vi "daq_TL Motor3DScan_initial2.vi"() -> ()   [LabVIEW 2014]
doc: "2D motor scan example Vi."
panel:
  in  "Z0 (33)":sgl format="%.3f"
  in  "X0 (34)":sgl=8.1 format="%.3f"
  in  "Y0 (32)":sgl=7.5 format="%.3f"
  out "Picture":picture
  out "Scale Z":sgl=0.1 format="%.3f"
  in  "Num Of Steps Z":i32=2
  out "MG17Motor C":dbl
  in  "Channel C":i32
  in  "Motor HWSerialNum C":u32=90834933
  in  "MG17Motor C":refnum<k7>(container)
  out "unsigned 8bit integer":u8[][](array[numeric])
  out "DAQ":dbl[][](array[numeric])
  out "Y":dbl[](array[numeric])
  out "Waveform Graph":waveform(dbl)(graph)
  out "dt":dbl
  out "t0":timestamp
  out "MG17Motor A":dbl
  out "MG17Motor B":dbl
  in  "Motor HWSerialNum B":u32=90834934
  in  "MG17Motor B":refnum<k7>(container)
  in  "MG17Motor A":refnum<k7>(container)
  in  "Num Of Steps X Y":i32=2
  out "Scale X Y":sgl=0.1 format="%.3f"
  in  "Both Channels":i32=10
  in  "Channel B":i32
  in  "Channel A":i32
  out "error":errorcluster
  in  "Motor HWSerialNum A":u32=90834932
  # "MG17Motor B\n (Y)"
  # "MG17Motor A\n (X)"
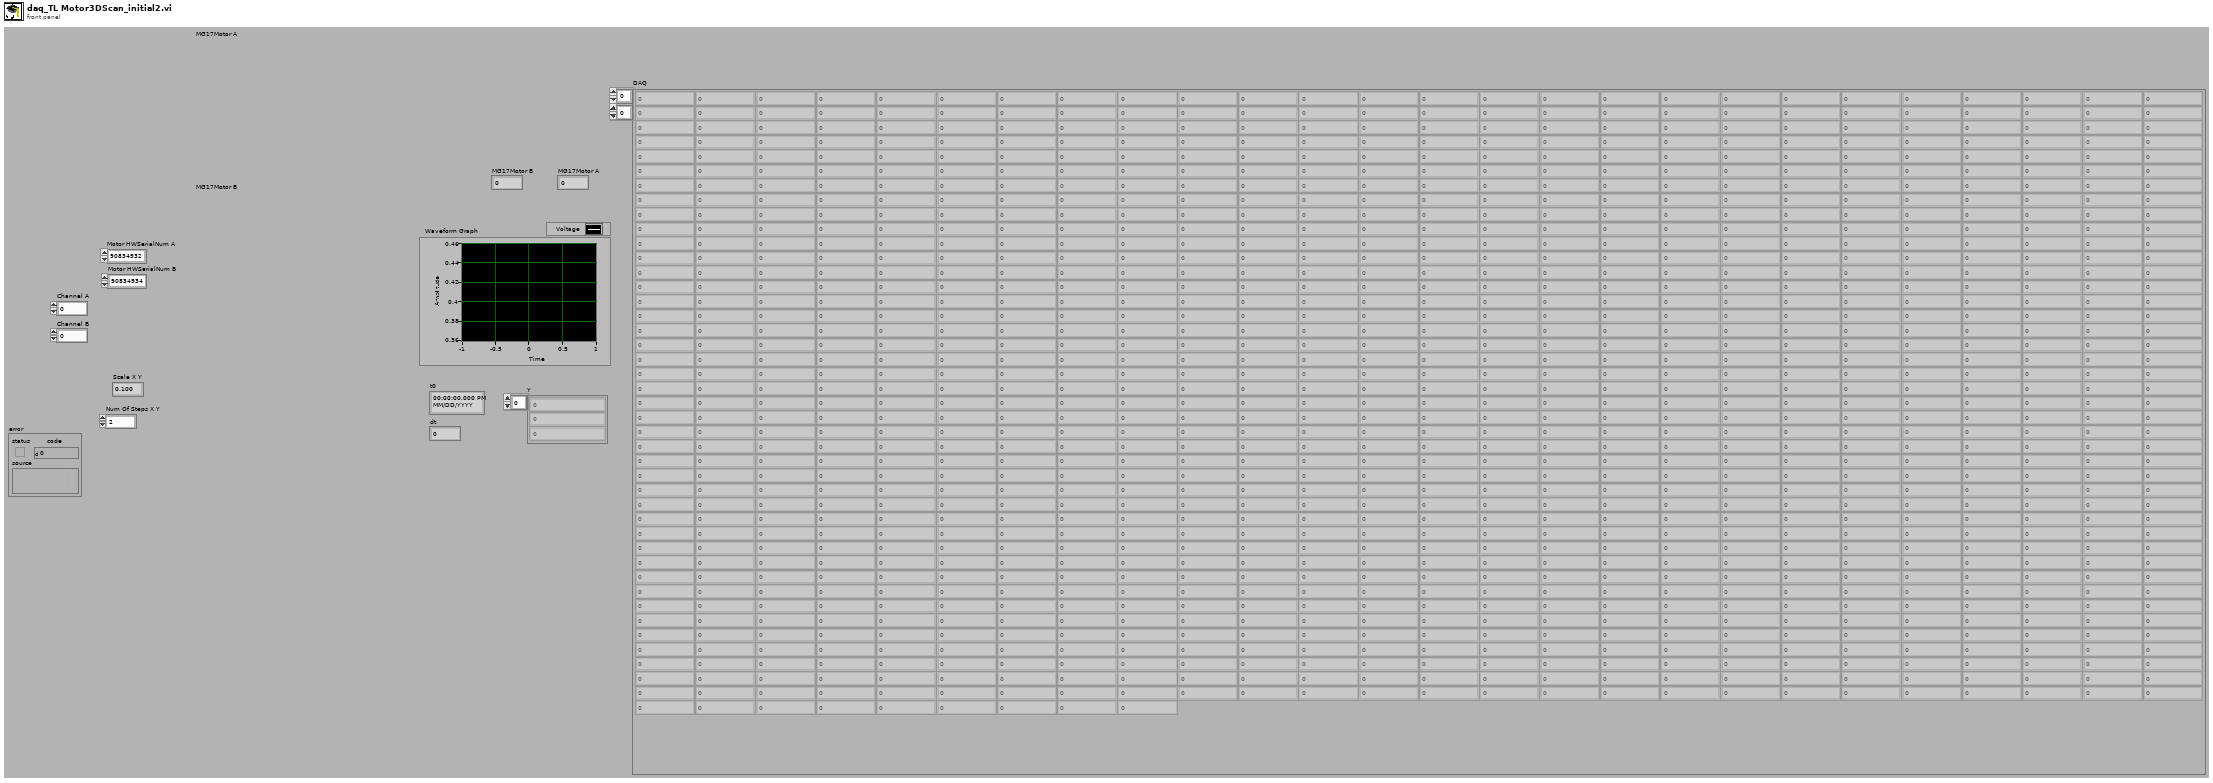
[diagram p1: front panel]
types:
  T1 = typedef "imagedata.ctl" = cluster{"image type":i32, "image depth":i32, "image":u8[], "mask":u8[], "colors":u32[], "Rectangle":cluster{"left":i16, "top":i16, "right":i16, "bottom":i16}}
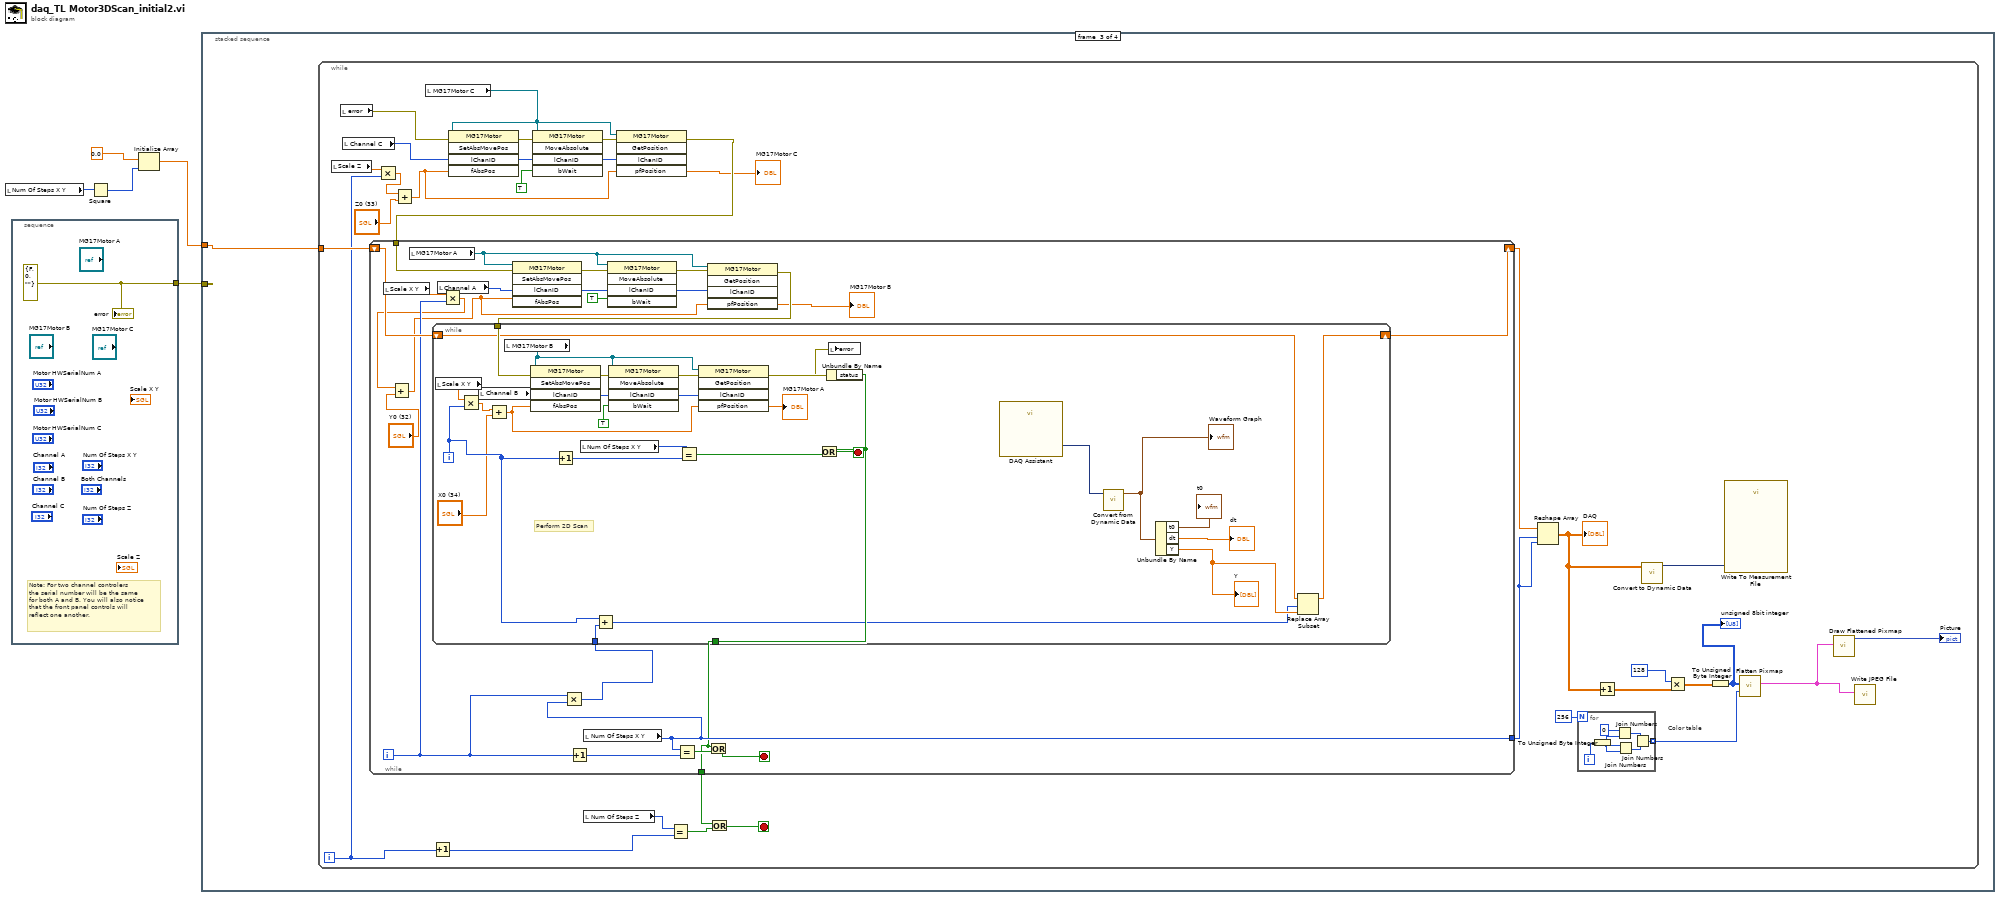
[diagram p0: block diagram]
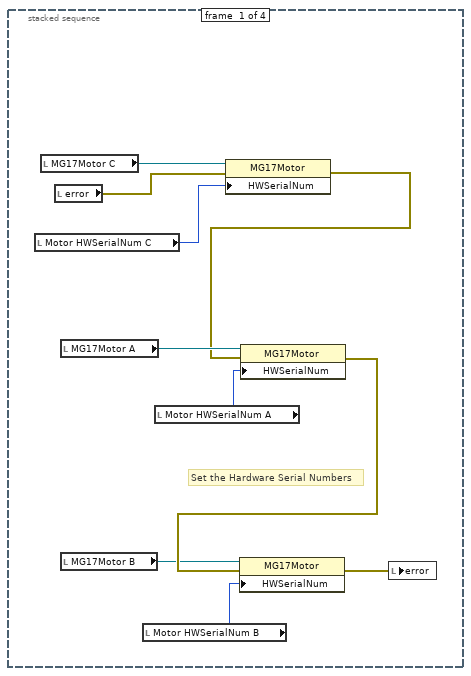
[diagram p2: hidden frame]
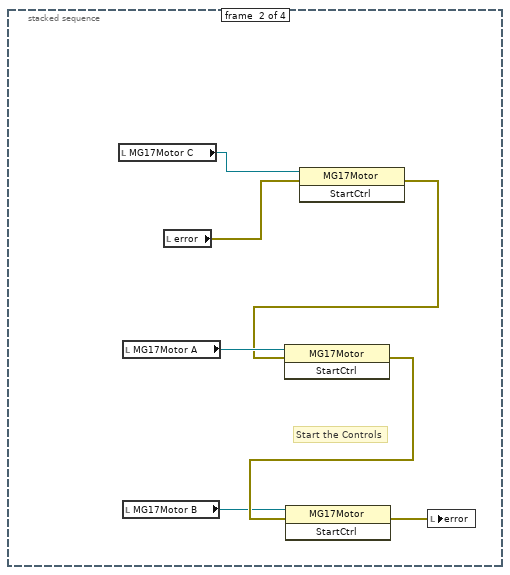
[diagram p3: hidden frame]
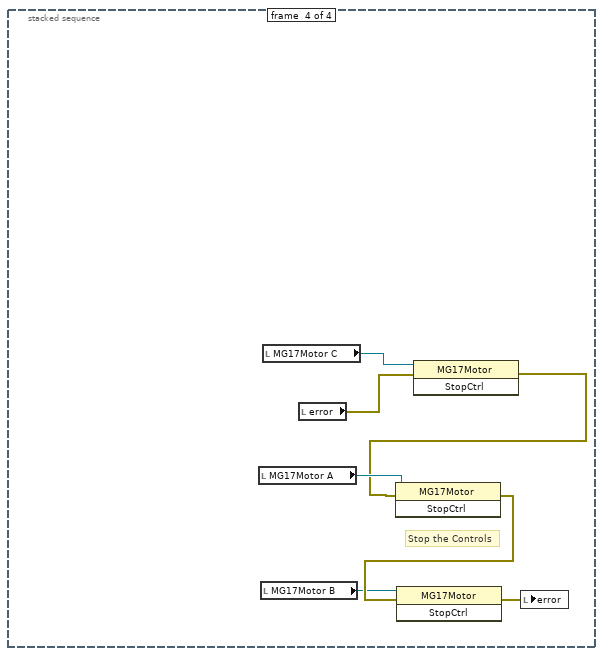
[diagram p4: hidden frame]
diagram:
  n1 = local read "Num Of Steps X Y"() -> (w1:i32)
  n2 = stacked-sequence {
    tunnel: [w6] -> w5
    frame #0 {
      w6 = errorcluster {"status"=FALSE, "code"=0, "source"=""} ("error in (no error)")
      # "Note: For two channel controlers\nthe serial number will be the same\nfor both A and B. You will also notice\nthat the front panel controls will\nreflect one another."
      "error" <- w6
    }
  }
  n3 = Square(x=w1) -> (x^2=w2:i32)
  n4 = Initialize Array(0.0, w2) -> (w3:dbl[])
  n5 = stacked-sequence {
    tunnel: w5 -> [_ _ _ _]
    tunnel: w3 -> [_ _ w24 _]
    frame #0 {
      # "Set the Hardware Serial Numbers"
      n6 = local read "Motor HWSerialNum C"() -> (w7:u32)
      n7 = local read "MG17Motor C"() -> (w10:refnum<k7>)
      n8 = local read "error"() -> (w9:errorcluster)
      n9 = local read "MG17Motor A"() -> (w15:refnum<k7>)
      n10 = local read "MG17Motor B"() -> (w12:refnum<k7>)
      n11 = local read "Motor HWSerialNum B"() -> (w11:u32)
      n12 = local read "Motor HWSerialNum A"() -> (w16:u32)
      n13 = property class="MG17Motor"(reference=w10, error in=w9, "HWSerialNum"=w7) -> (error out=w8:errorcluster)  [unwired: 1 out]
      n14 = property class="MG17Motor"(reference=w15, error in=w8, "HWSerialNum"=w16) -> (error out=w14:errorcluster)  [unwired: 1 out]
      n15 = property class="MG17Motor"(reference=w12, error in=w14, "HWSerialNum"=w11) -> (error out=w13:errorcluster)  [unwired: 1 out]
      n16 = local write "error"(w13) -> ()
    }
    frame #1 {
      # "Start the Controls"
      n17 = local read "MG17Motor C"() -> (w17:refnum<k7>)
      n18 = local read "MG17Motor A"() -> (w23:refnum<k7>)
      n19 = local read "MG17Motor B"() -> (w20:refnum<k7>)
      n20 = local read "error"() -> (w19:errorcluster)
      n21 = invoke class="MG17Motor" method="StartCtrl"(reference=w17, error in=w19) -> (error out=w18:errorcluster)  [unwired: 1 in, 2 out]
      n22 = invoke class="MG17Motor" method="StartCtrl"(reference=w23, error in=w18) -> (error out=w21:errorcluster)  [unwired: 1 in, 2 out]
      n23 = invoke class="MG17Motor" method="StartCtrl"(reference=w20, error in=w21) -> (error out=w22:errorcluster)  [unwired: 1 in, 2 out]
      n24 = local write "error"(w22) -> ()
    }
    frame #2 {
      n25 = while {
        tunnel: w24 -> [w56]
        i -> [w33]
        stop <- w35 stop-if-true
        # "Color table"
        # "Perform 2D Scan"
        n26 = local read "Scale Z"() -> (w34:sgl)
        n27 = local read "error"() -> (w42:errorcluster)
        n28 = local read "Channel C"() -> (w32:i32)
        n29 = Multiply(x=w34, y=w33) -> (x*y=w28:sgl)
        n30 = Add(x=w28, y="Z0 (33)") -> (x+y=w27:sgl)
        n31 = local read "MG17Motor C"() -> (w39:refnum<k7>)
        n32 = Increment(x=w33) -> (x+1=w29:i32)
        n33 = invoke class="MG17Motor" method="SetAbsMovePos"(reference=w39, error in=w42, "lChanID"=w32, "fAbsPos"=w27) -> (error out=w46:errorcluster, "lChanID"=w45:i32)  [unwired: 1 in, 3 out]
        n34 = invoke class="MG17Motor" method="MoveAbsolute"(reference=w39, error in=w46, "lChanID"=w45, "bWait"=TRUE) -> (error out=w41:errorcluster, "lChanID"=w43:i32)  [unwired: 1 in, 3 out]
        n35 = while {
          shift-right: [w72] -> w51
          shift-left: w56 -> [w73]
          tunnel: [w69] -> w55
          tunnel: w41 -> [w68]
          tunnel: [w67] -> w38
          i -> [w70]
          stop <- w79 stop-if-true
          n36 = local read "Scale X Y"() -> (w85:sgl)
          n37 = local read "MG17Motor A"() -> (w77:refnum<k7>)
          n38 = local read "Channel A"() -> (w66:i32)
          n39 = Multiply(x=w85, y=w70) -> (x*y=w64:sgl)
          n40 = Add(x=w64, y="Y0 (32)") -> (x+y=w63:sgl)
          n41 = invoke class="MG17Motor" method="SetAbsMovePos"(reference=w77, error in=w68, "lChanID"=w66, "fAbsPos"=w63) -> (error out=w84:errorcluster, "lChanID"=w83:i32)  [unwired: 1 in, 3 out]
          n42 = Increment(x=w70) -> (x+1=w80:i32)
          n43 = local read "Num Of Steps X Y"() -> (w69:i32)
          n44 = Multiply(x=w70, y=w69) -> (x*y=w71:i32)
          n45 = invoke class="MG17Motor" method="MoveAbsolute"(reference=w77, error in=w84, "lChanID"=w83, "bWait"=TRUE) -> (error out=w76:errorcluster, "lChanID"=w75:i32)  [unwired: 1 in, 3 out]
          n46 = Equal?(x=w69, y=w80) -> (x = y?=w81:bool)
          n47 = invoke class="MG17Motor" method="GetPosition"(reference=w77, error in=w76, "lChanID"=w75, "pfPosition"=w63) -> (error out=w78:errorcluster, "pfPosition"=→"MG17Motor B":sgl)  [unwired: 1 in, 3 out]
          n48 = while {
            tunnel: [w107] -> w67
            tunnel: w78 -> [w111]
            shift-right: [w94] -> w72
            shift-left: w73 -> [w96]
            tunnel: w71 -> [w92]
            i -> [w89]
            stop <- w105 stop-if-true
            n49 = local read "Scale X Y"() -> (w109:sgl)
            n50 = Multiply(x=w109, y=w89) -> (x*y=w87:sgl)
            n51 = local read "Channel B"() -> (w110:i32)
            n52 = Add(x=w87, y="X0 (34)") -> (x+y=w88:sgl)
            n53 = local read "MG17Motor B"() -> (w103:refnum<k7>)
            n54 = invoke class="MG17Motor" method="SetAbsMovePos"(reference=w103, error in=w111, "lChanID"=w110, "fAbsPos"=w88) -> (error out=w114:errorcluster, "lChanID"=w113:i32)  [unwired: 1 in, 3 out]
            n55 = Increment(x=w89) -> (x+1=w106:i32)
            n56 = local read "Num Of Steps X Y"() -> (w93:i32)
            n57 = Add(x=w89, y=w92) -> (x+y=w91:i32)
            n58 = invoke class="MG17Motor" method="MoveAbsolute"(reference=w103, error in=w114, "lChanID"=w113, "bWait"=TRUE) -> (error out=w102:errorcluster, "lChanID"=w101:i32)  [unwired: 1 in, 3 out]
            n59 = Equal?(x=w93, y=w106) -> (x = y?=w108:bool)
            n60 = invoke class="MG17Motor" method="GetPosition"(reference=w103, error in=w102, "lChanID"=w101, "pfPosition"=w88) -> (error out=w104:errorcluster, "pfPosition"=→"MG17Motor A":sgl)  [unwired: 1 in, 3 out]
            n61 = Unbundle By Name(w104) -> ("status"=w107:bool)
            n62 = Or(x=w107, y=w108) -> (x .or. y?=w105:bool)
            n63 = local write "error"(w102) -> ()
            n64 = call "DAQ Assistant"() -> ("data"=w90:dynamicdata)  [unwired: 17 in, 2 out]
            n65 = call "Convert from Dynamic Data"("Dynamic Data Type"=w90) -> ("Waveform"=w97:waveform(dbl))  [unwired: 3 in]
            "Waveform Graph" <- w97
            n66 = Unbundle By Name(w97) -> ("t0"=→"t0":timestamp, "dt"=→"dt":dbl, "Y"=w95:dbl[])
            "Y" <- w95
            n67 = Replace Array Subset(array=w96, new element=w95, index=w91) -> (w94:dbl[])
          }
          n68 = Or(x=w67, y=w81) -> (x .or. y?=w79:bool)
        }
        n69 = local read "Num Of Steps Z"() -> (w37:i32)
        n70 = invoke class="MG17Motor" method="GetPosition"(reference=w39, error in=w41, "lChanID"=w43, "pfPosition"=w27) -> ("pfPosition"=→"MG17Motor C":sgl)  [unwired: 1 in, 4 out]
        n71 = Equal?(x=w37, y=w29) -> (x = y?=w36:bool)
        n72 = Or(x=w38, y=w36) -> (x .or. y?=w35:bool)
        n73 = Reshape Array(w51, w55, w55) -> (w31:dbl[][])
        "DAQ" <- w31
        n74 = for {
          N: 256 -> [_]
          tunnel: [w57] -> w52 mode=indexing
          i -> [w62]
          n75 = To Unsigned Byte Integer(number=w62) -> (unsigned 8bit integer=w61:u8)
          n76 = Join Numbers(hi=u8 0, lo=w61) -> ((hi.lo)=w59:u16)
          n77 = Join Numbers(hi=w61, lo=w61) -> ((hi.lo)=w58:u16)
          n78 = Join Numbers(hi=w59, lo=w58) -> ((hi.lo)=w57:u32)
        }
        n79 = Increment(x=w31) -> (x+1=w47:dbl[][])
        n80 = call "Convert to Dynamic Data"("2D Array"=w31) -> ("Dynamic Data Type"=w30:dynamicdata)  [unwired: 3 in]
        n81 = Multiply(x=128, y=w47) -> (x*y=w48:dbl[][])
        n82 = To Unsigned Byte Integer(number=w48) -> (unsigned 8bit integer=w50:u8[][])
        "unsigned 8bit integer" <- w50
        n83 = call "Write To Measurement File"("Signals"=w30) -> ()  [unwired: 16 in, 3 out]
        n84 = call <vilib>:"Flatten Pixmap.vi"("colors"=w52, "8-bit pixmap"=w50) -> ("image data"=w25:T1)  [unwired: 9 in]
        n85 = call <vilib>:"Draw Flattened Pixmap.vi"("image data"=w25) -> ("new picture"=→"Picture":picture)  [unwired: 8 in]
        n86 = call <vilib>:"Write JPEG File.vi"("image data"=w25) -> ()  [unwired: 9 in, 2 out]
      }
    }
    frame #3 {
      # "Stop the Controls"
      n87 = local read "MG17Motor A"() -> (w121:refnum<k7>)
      n88 = local read "MG17Motor B"() -> (w118:refnum<k7>)
      n89 = local read "MG17Motor C"() -> (w115:refnum<k7>)
      n90 = local read "error"() -> (w117:errorcluster)
      n91 = invoke class="MG17Motor" method="StopCtrl"(reference=w115, error in=w117) -> (error out=w116:errorcluster)  [unwired: 1 in, 2 out]
      n92 = invoke class="MG17Motor" method="StopCtrl"(reference=w121, error in=w116) -> (error out=w120:errorcluster)  [unwired: 1 in, 2 out]
      n93 = invoke class="MG17Motor" method="StopCtrl"(reference=w118, error in=w120) -> (error out=w119:errorcluster)  [unwired: 1 in, 2 out]
      n94 = local write "error"(w119) -> ()
    }
  }
